vi "sequence util_edit.vi"(8 "error in":errorcluster, 9 "Sequence Array":string[](array[string])=["----------    AH Bridge: Save GPIB address   ", "Write to VISA, GPIB::27::INSTR, FILE STORE GPIB USERPON", "----------    LakeShore 340 controller: change heater power (0-5, 0: off)  ", "Write to VISA, GPIB::12::INSTR, RANGE 0", "----------    Scheduled T-control for the He3 system   ", "Wait for 12 hour", "Set Temperature LS336 ( GPIB0::12::INSTR ) 45 K at 0 K/min, Output 1", "Wait for 60 s", "Wait for Temperature Less than 1.8 K Sensor C of LS336 ( GPIB0::14::INSTR ) Timeout 30 min", "Wait for 60 min", "Set Temperature LS336 ( GPIB0::12::INSTR ) 0.1 K at 0 K/min, Output 1", "----------    Motor control (use Instrumet:Set:MotorControl command structure)  ", "Set MotorControl ( BLM ) 12345 0.2", "Wait for VI value localhost, BLM_ManualControl.vi, BLM Position, Within, 12345, 10 min", "Wait for 10 s", "END SEQUENCE"]) -> (0 "error out":errorcluster, 1 "Item Names out":string[](array[string]))   [LabVIEW 2020]
panel:
  in  "Edit panel":string
  in  "highlight line contains following text":cluster{"String":string, "Color Box":u32}[](array[cluster])
  in  "file (use dialog)":path
  in  "expand macro":bool
  in  "Disply panel":i32(listbox)
  in  "Cancel":bool
  in  "Done":bool
  # "(can be edited)"
  # "(can be edited using internal or external editor)"
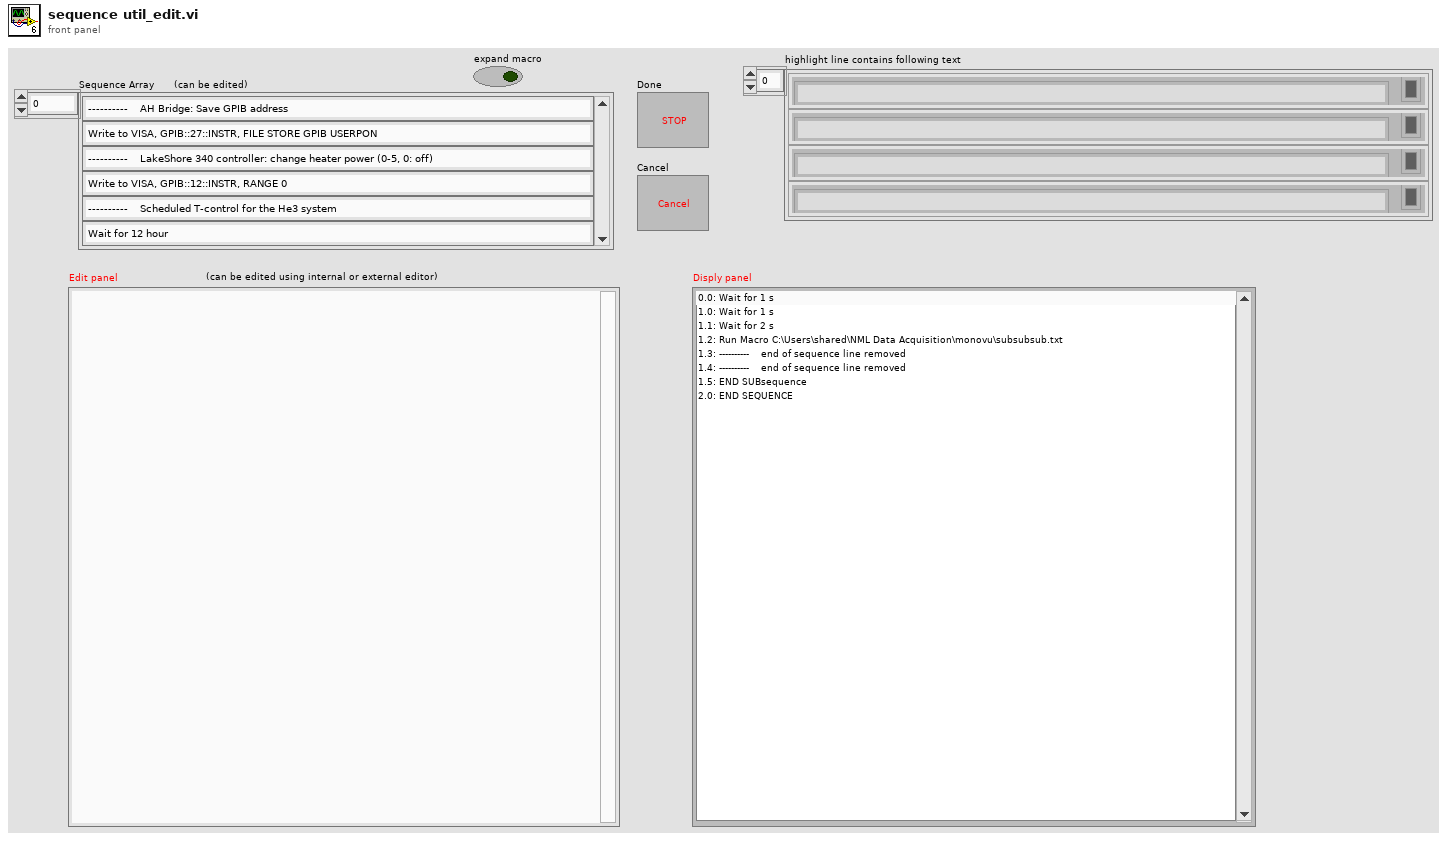
[diagram p1: front panel]
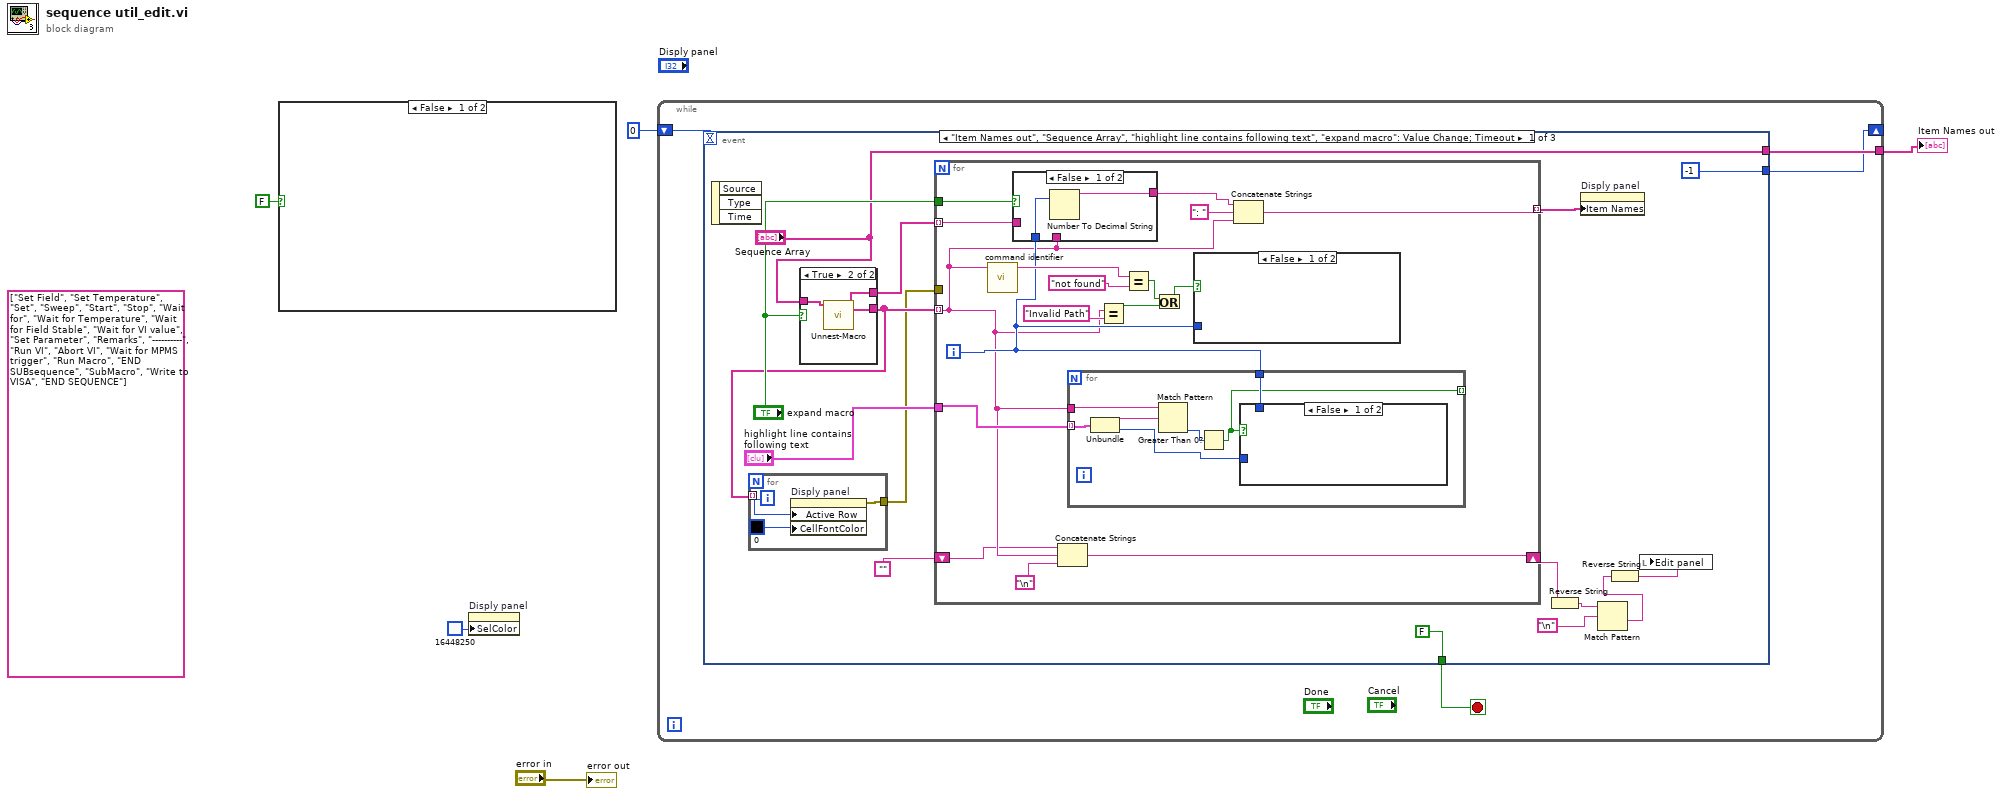
[diagram p0: block diagram]
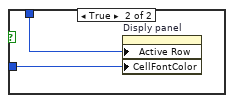
[diagram p3: hidden frame]
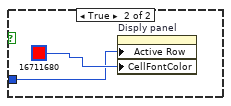
[diagram p5: hidden frame]
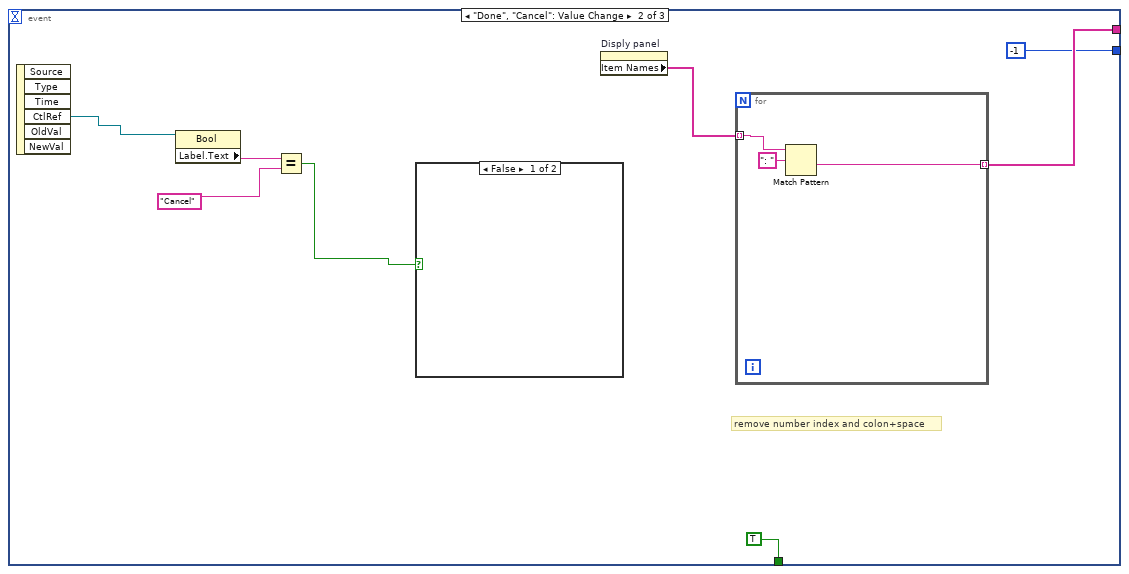
[diagram p6: hidden frame]
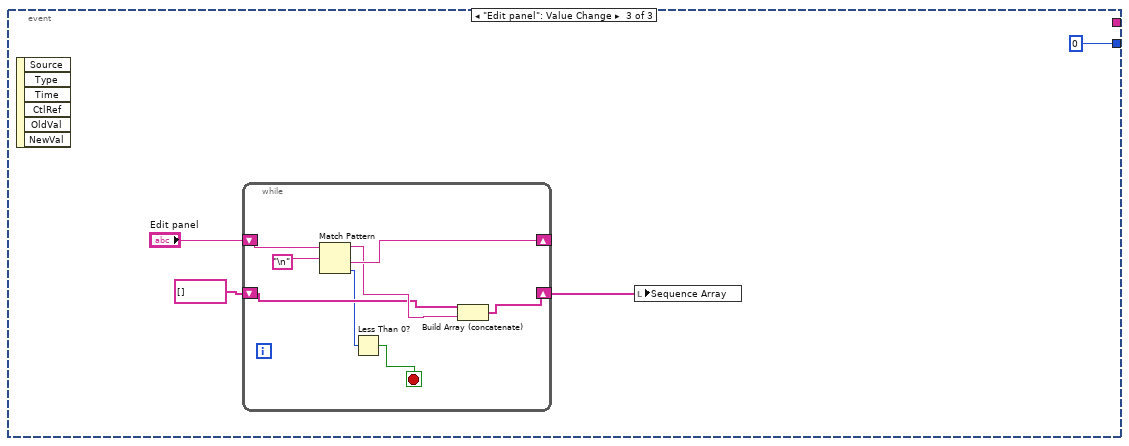
[diagram p8: hidden frame]
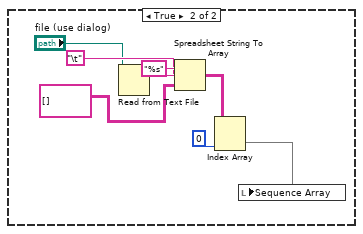
[diagram p9: hidden frame]
diagram:
  (unwired) string[] ["Set Field", "Set Temperature", "Set", "Sweep", "Start", "Stop", "Wait for", "Wait for Temperature", "Wait for Field Stable", "Wait for VI value", "Set Parameter", "Remarks", "----------", "Run VI", "Abort VI", "Wait for MPMS trigger", "Run Macro", "END SUBsequence", "SubMacro", "Write to VISA", "END SEQUENCE"] ("command list-all")
  n1 = case shown="False" FALSE {
    frame False {
    }
    frame True {
      n2 = Read from Text File(file (use dialog)="file (use dialog)") -> (text=w13:string)  [unwired: 3 in, 3 out]
      n3 = Spreadsheet String To Array(delimiter (Tab)="\t", format string="%s", spreadsheet string=w13, array type (2D Dbl)=string[][] []) -> (array=w10:string[][])
      n4 = Index Array(array=w10, index (col)=0 ("index (row)")) -> (element=w7:string[])  [unwired: 1 in]
      n5 = local write "Sequence Array"(w7) -> ()
    }
  }
  n6 = property on="Disply panel" class="LstBox (strict)"("SelColor"=u32 16448250 ("Selection Color")) -> ()  [unwired: 2 in, 2 out]
  n7 = while {
    shift-right: [w14] -> _
    shift-left: 0 ("sequence in") -> [w16]
    tunnel: [w15] -> w2
    stop <- w17 stop-if-true
    n8 = event shown="[0] \"Item Names out\", \"Sequence Array\", \"highlight line contains following text\", \"expand macro\": Value Change;  Timeout" {
      selector: _ -> [_ _ _]
      dyn-events: _ -> [_ _ _]
      timeout: w16 -> [_ _ _]
      tunnel: [FALSE TRUE _] -> w17
      tunnel: ["Sequence Array" w72 _] -> w15
      tunnel: [-1 ("sequence in") -1 ("sequence in") 0 ("sequence in")] -> w14
      event "Item Names out", "Sequence Array", "highlight line contains following text", "expand macro": Value Change; Timeout {
        n9 = event-data() -> ()  [unwired: 1 in, 3 out]
        n10 = case shown="True" "expand macro" {
          tunnel: "Sequence Array" -> [w36 w39]
          tunnel: [w36 w38] -> w27
          tunnel: [w36 w37] -> w28
          frame False {
          }
          frame True {
            n11 = call "Unnest-Macro.vi"("Item Names IN"=w39) -> ("unnested items"=w38:string[], "item index"=w37:string[])  [unwired: 9 in]
          }
        }
        n12 = for {
          tunnel: w27 -> [_] mode=indexing
          tunnel: [w33] -> w26
          i -> [w35]
          n13 = property on="Disply panel" class="LstBox (strict)"("Active Row"=w35, "CellFontColor"=u32 0 ("Active Row:Cell Font:Color")) -> (error out=w33:errorcluster)  [unwired: 2 in, 1 out]
        }
        n14 = for {
          tunnel: w27 -> [w43] mode=indexing
          tunnel: [w51] -> w31 mode=indexing
          tunnel: w28 -> [w54] mode=indexing
          tunnel: "expand macro" -> [w53]
          tunnel: "highlight line contains following text" -> [w49]
          tunnel: w26 -> [_]
          shift-right: [w40] -> w19
          shift-left: "" -> [w41]
          i -> [w48]
          n15 = call "command identifier.vi"("Input command"=w43) -> ("Identifield command"=w55:string)  [unwired: 10 in]
          n16 = case shown="False" w53 {
            tunnel: [w67 w68] -> w50
            tunnel: w48 -> [w66 _]
            tunnel: w54 -> [_ w68]
            tunnel: w43 -> [_ _]
            frame False {
              n17 = Number To Decimal String(number=w66) -> (decimal integer string=w67:string)  [unwired: 1 in]
            }
            frame True {
            }
          }
          n18 = Concatenate Strings(w41, w43, "\n") -> (w40:string)
          n19 = for {
            tunnel: w49 -> [w61] mode=indexing
            tunnel: w43 -> [w63]
            tunnel: w48 -> [w58]
            tunnel: [w57] -> _ mode=indexing
            n20 = Unbundle(w61) -> ("String"=w60:string, "Color Box"=w59:u32)
            n21 = Match Pattern(string=w63, regular expression=w60) -> (offset past match=w62:i32)  [unwired: 1 in, 3 out]
            n22 = Greater Than 0?(x=w62) -> (x > 0?=w57:bool)
            n23 = case shown="False" w57 {
              tunnel: w59 -> [_ w64]
              tunnel: w58 -> [_ w65]
              frame False {
              }
              frame True {
                n24 = property on="Disply panel" class="LstBox (strict)"("Active Row"=w65, "CellFontColor"=w64) -> ()  [unwired: 2 in, 2 out]
              }
            }
          }
          n25 = Equal?(x=w43, y="Invalid Path") -> (x = y?=w45:bool)
          n26 = Equal?(x=w55, y="not found") -> (x = y?=w46:bool)
          n27 = Or(x=w46, y=w45) -> (x .or. y?=w44:bool)
          n28 = case shown="False" w44 {
            tunnel: w48 -> [_ w69]
            frame False {
            }
            frame True {
              n29 = property on="Disply panel" class="LstBox (strict)"("Active Row"=w69, "CellFontColor"=u32 16711680 ("Active Row:Cell Font:Color")) -> ()  [unwired: 2 in, 2 out]
            }
          }
          n30 = Concatenate Strings(w50, ": ", w43) -> (w51:string)
        }
        n31 = Reverse String(1:w19) -> (0:w21:string)
        n32 = property on="Disply panel" class="LstBox (strict)"("Item Names"=w31) -> ()  [unwired: 2 in, 2 out]
        n33 = Match Pattern(string=w21, regular expression="\n") -> (after substring=w22:string)  [unwired: 1 in, 3 out]
        n34 = Reverse String(1:w22) -> (0:w18:string)
        n35 = local write "Edit panel"(w18) -> ()
      }
      event "Done", "Cancel": Value Change {
        # "remove number index and colon+space"
        n36 = event-data() -> ("CtlRef"=w77:refnum<vi>)  [unwired: 1 in, 5 out]
        n37 = property class="Bool"(reference=w77) -> ("Label.Text"=w76:string)  [unwired: 1 in, 2 out]
        n38 = Equal?(x=w76, y="Cancel") -> (x = y?=w74:bool)
        n39 = case shown="False" w74 {
          frame False {
          }
          frame True {
          }
        }
        n40 = property on="Disply panel" class="LstBox (strict)"() -> ("Item Names"=w73:string[])  [unwired: 2 in, 2 out]
        n41 = for {
          tunnel: w73 -> [w81] mode=indexing
          tunnel: [w79] -> w72 mode=indexing
          n42 = Match Pattern(string=w81, regular expression=": ") -> (after substring=w79:string)  [unwired: 1 in, 3 out]
        }
      }
      event "Edit panel": Value Change {
        n43 = event-data() -> ()  [unwired: 1 in, 6 out]
        n44 = while {
          shift-right: [w91] -> _
          shift-left: "Edit panel" -> [w93]
          shift-right: [w89] -> w82
          shift-left: string[] [] -> [w88]
          stop <- w86 stop-if-true
          n45 = Match Pattern(string=w93, regular expression="\n") -> (before substring=w90:string, after substring=w91:string, offset past match=w87:i32)  [unwired: 1 in, 1 out]
          n46 = Less Than 0?(x=w87) -> (x < 0?=w86:bool)
          n47 = Build Array (concatenate)(w88, w90) -> (w89:string[])
        }
        n48 = local write "Sequence Array"(w82) -> ()
      }
    }
  }
  "Item Names out" <- w2
  "error out" <- "error in"
